vi "Get Plot Data.vi"(8 "error in (no error)":errorcluster, 11 "NI_Robotics_Serial Robot Arm in":refnum<class "NI_Robotics_Serial Robot Arm.lvclass">) -> (0 "error out":errorcluster, 1 "Serial Arm Scene":refnum<vi>, 2 "Plot Data":T1[](array[typedef]), 3 "NI_Robotics_Serial Robot Arm out":refnum<class "NI_Robotics_Serial Robot Arm.lvclass">, 4 "Scale":dbl)   [LabVIEW 2017, in "NI_Robotics_Serial Robot Arm.lvclass"]
uses:
  <vilib>/robotics/Kinematics/Robot/NI_Robotics_Serial Robot Arm.lvclass
  <vilib>/robotics/Kinematics/Plotting/Joint Control.ctl
  <vilib>/robotics/Kinematics/Plotting/Joint Type.ctl
  <vilib>/robotics/Kinematics/Robot/NI_Robotics_Serial Robot Arm.lvclass/NI_Robotics_Serial Robot Arm.ctl
  <vilib>/robotics/Kinematics/Plotting/NI_Robotics_3DKinematics.lvlib
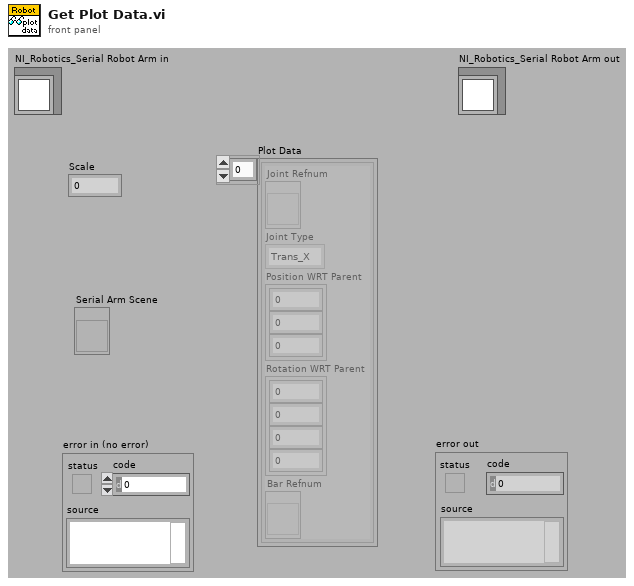
[diagram p1: front panel]
types:
  T1 = typedef "NI_Robotics_3DKinematics.lvlib/Joint Control.ctl" = cluster{"Joint Refnum":refnum<vi>, "Joint Type":T2, "Position WRT Parent":dbl[], "Rotation WRT Parent":dbl[], "Bar Refnum":refnum<vi>}
  T2 = typedef "NI_Robotics_3DKinematics.lvlib/Joint Type.ctl" = enum16{"Trans_X", "Trans_Y", "Trans_Z", "Rot_X", "Rot_Y", "Rot_Z", "None"}
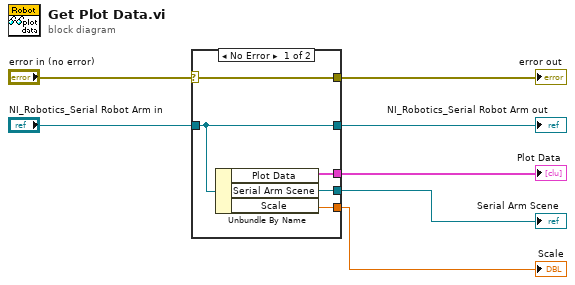
[diagram p0: block diagram]
diagram:
  n1 = case shown="No Error" "error in (no error)" {
    selector: "error in (no error)" -> [w12 w13]
    tunnel: [w12 w13] -> w6
    tunnel: [w11 w14] -> w4
    tunnel: "NI_Robotics_Serial Robot Arm in" -> [w11 w14]
    tunnel: [w10 _] -> w3
    tunnel: [w9 _] -> w2
    tunnel: [w8 _] -> w1
    frame No Error {
      n2 = Unbundle By Name(w11) -> ("Plot Data"=w10:T1[], "Serial Arm Scene"=w9:refnum<vi>, "Scale"=w8:dbl)
    }
    frame Error {
    }
  }
  "error out" <- w6
  "NI_Robotics_Serial Robot Arm out" <- w4
  "Plot Data" <- w3
  "Serial Arm Scene" <- w2
  "Scale" <- w1
